vi "PH_4_Pos_Selector.PC Define Position.vi"(0 "VI in":refnum<vi>, 5 "error in (no error)":errorcluster) -> (14 "VI out":refnum<vi>, 19 "error out":errorcluster)   [LabVIEW 2014, in "PH_4_Pos_Selector.lvlib"]
uses:
  PH_4_Pos_Selector.lvlib
  PH_Basics/PH_AxisGUI_BaseClass/PH_AxisGUI_BaseClass.lvlib
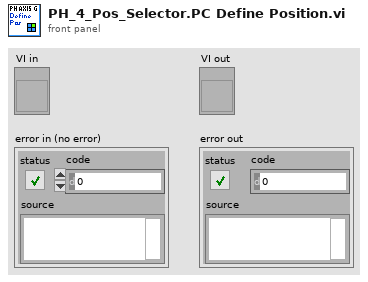
[diagram p1: front panel]
types:
  T1 = typedef "PH_4_Pos_Selector.lvlib/PH_4_Pos_Selector.i attribute.ctl" = cluster{"GUI Refs":cluster{"Position I":refnum<vi>, "Position II":refnum<vi>, "Position III":refnum<vi>, "Position IV":refnum<vi>, "rel. Mode?":refnum<vi>, "Define Selector":refnum<vi>}, "Current Position":T2, "Service ID Position":i32, "Position Array":T3[], "Description Array":string[], "relative Mode":bool, "Wanted Define Selector Position":string}
  T2 = typedef "PH_4_Pos_Selector.lvlib/PH_4_Pos_Selector.Position Selector.ctl" = u16
  T3 = typedef "PH_4_Pos_Selector.lvlib/PH_4_Pos_Selector.Position.ctl" = cluster{"Axis 1":dbl, "Axis 2":dbl}
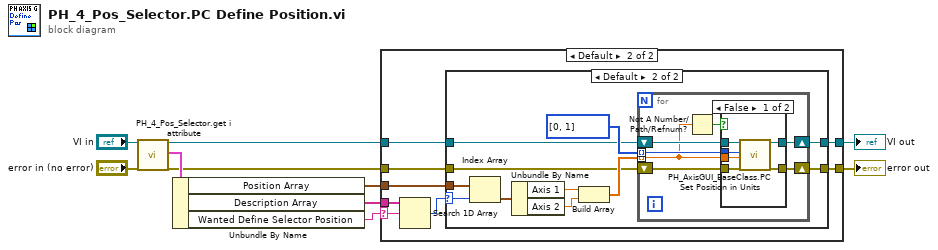
[diagram p0: block diagram]
diagram:
  n1 = call "PH_4_Pos_Selector.get i attribute.vi"("i ref in"="VI in", "error in (no error)"="error in (no error)") -> ("i ref out"=w8:refnum<vi>, "i attribute"=w9:T1, "error out"=w7:errorcluster)  [unwired: 15 in]
  n2 = Unbundle By Name(w9) -> ("Position Array"=w10:T3[], "Description Array"=w2:string[], "Wanted Define Selector Position"=w1:string)
  n3 = case shown="Default" w1 {
    selector: w1 -> [_ w13]
    tunnel: w10 -> [_ w20]
    tunnel: w8 -> [w12 w19]
    tunnel: w7 -> [w11 w18]
    tunnel: [w11 w17] -> w4
    tunnel: [w12 w16] -> w3
    tunnel: w2 -> [_ w15]
    frame "False" {
    }
    frame Default {
      n4 = Search 1D Array(1D array=w15, element=w13) -> (index of element=w14:i32)  [unwired: 1 in]
      n5 = case shown="Default" w14 {
        selector: w14 -> [_ w23]
        tunnel: w20 -> [_ w28]
        tunnel: w19 -> [w22 w27]
        tunnel: w18 -> [w21 w26]
        tunnel: [w21 w25] -> w17
        tunnel: [w22 w24] -> w16
        frame -1 {
        }
        frame Default {
          n6 = Index Array(array=w28, index=w23) -> (element=w29:T3)
          n7 = Unbundle By Name(w29) -> ("Axis 1"=w30:dbl, "Axis 2"=w31:dbl)
          n8 = Build Array(w30, w31) -> (w32:dbl[])
          n9 = for {
            shift-right: [w37] -> w25
            shift-left: w26 -> [w40]
            shift-right: [w38] -> w24
            shift-left: w27 -> [w39]
            tunnel: w32 -> [w35] mode=indexing
            tunnel: i32[] [0, 1] -> [w36] mode=indexing
            n10 = Not A Number/Path/Refnum?(number/path/refnum=w35) -> (NaN/Path/Refnum?=w34:bool)
            n11 = case shown="False" w34 {
              tunnel: w40 -> [w46 w47]
              tunnel: w39 -> [w45 w48]
              tunnel: [w44 w48] -> w38
              tunnel: [w43 w47] -> w37
              tunnel: w36 -> [w42 _]
              tunnel: w35 -> [w41 _]
              frame False {
                n12 = call "PH_AxisGUI_BaseClass.PC Set Position in Units.vi"("VI in"=w45, "Axis"=w42, "Position to set [Units]"=w41, "error in (no error)"=w46) -> ("VI out"=w44:refnum<vi>, "error out"=w43:errorcluster)  [unwired: 14 in]
              }
              frame True {
              }
            }
          }
        }
      }
    }
  }
  "error out" <- w4
  "VI out" <- w3
